vi "Receive.vi"(10 "MessageBuffer":T1, 11 "Clear?":bool) -> (2 "Receive":string[][](array[string]))   [LabVIEW 2020]
panel:
  out "error out":errorcluster caption="错误输出"
  in  "error in":errorcluster caption="错误输入"
  # "Receive"
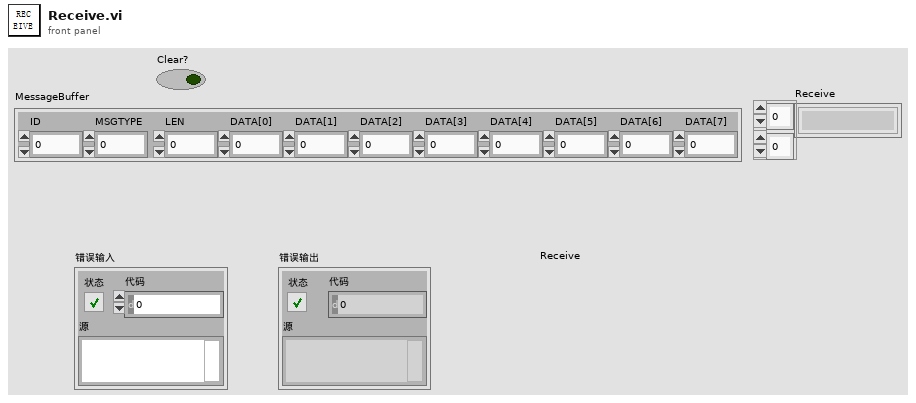
[diagram p1: front panel]
types:
  T1 = cluster{"ID":u32, "MSGTYPE":u8, "LEN":u8, "DATA[0]":u8, "DATA[1]":u8, "DATA[2]":u8, "DATA[3]":u8, "DATA[4]":u8, "DATA[5]":u8, "DATA[6]":u8, "DATA[7]":u8}
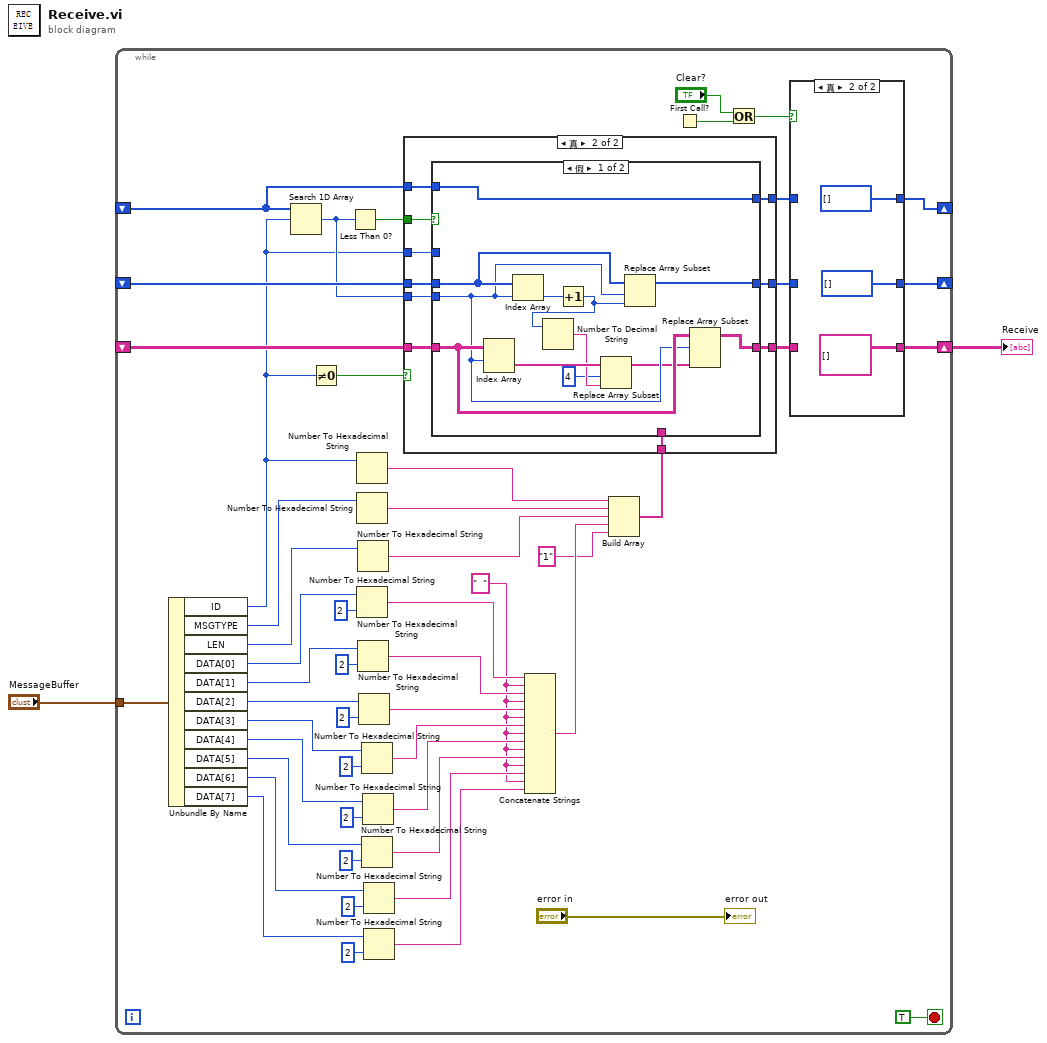
[diagram p0: block diagram]
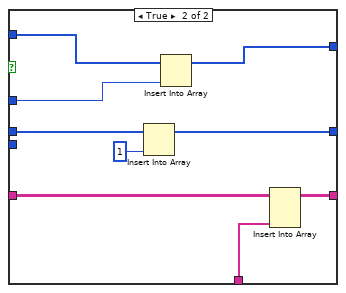
[diagram p3: hidden frame]
diagram:
  n1 = while {
    tunnel: "MessageBuffer" -> [w54]
    shift-right: [w20] -> _
    shift-left: _ -> [w6]
    shift-right: [w19] -> _
    shift-left: _ -> [w17]
    shift-right: [w14] -> w1
    shift-left: _ -> [w13]
    stop <- TRUE stop-if-true
    w27 = "  "
    n2 = Unbundle By Name(w54) -> ("ID"=w4:u32, "MSGTYPE"=w53:u8, "LEN"=w52:u8, "DATA[0]"=w51:u8, "DATA[1]"=w48:u8, "DATA[2]"=w46:u8, "DATA[3]"=w44:u8, "DATA[4]"=w42:u8, "DATA[5]"=w38:u8, "DATA[6]"=w37:u8, "DATA[7]"=w36:u8)
    n3 = Search 1D Array(1D array=w6, element=w4) -> (index of element=w15:i32)  [unwired: 1 in]
    n4 = Not Equal To 0?(x=w4) -> (x != 0?=w3:bool)
    n5 = Less Than 0?(x=w15) -> (x < 0?=w18:bool)
    n6 = Number To Hexadecimal String(2:w4) -> (0:w26:string)  [unwired: 1 in]
    n7 = Number To Hexadecimal String(2:w53) -> (0:w25:string)  [unwired: 1 in]
    n8 = Number To Hexadecimal String(1:i16 2 ("宽度(-)"), 2:w51) -> (0:w35:string)
    n9 = Number To Hexadecimal String(2:w52) -> (0:w24:string)  [unwired: 1 in]
    n10 = Number To Hexadecimal String(1:i16 2 ("宽度(-)"), 2:w48) -> (0:w34:string)
    n11 = Number To Hexadecimal String(1:i16 2 ("宽度(-)"), 2:w46) -> (0:w33:string)
    n12 = Number To Hexadecimal String(1:i16 2 ("宽度(-)"), 2:w44) -> (0:w32:string)
    n13 = Number To Hexadecimal String(1:i16 2 ("宽度(-)"), 2:w38) -> (0:w30:string)
    n14 = Number To Hexadecimal String(1:i16 2 ("宽度(-)"), 2:w42) -> (0:w31:string)
    n15 = Number To Hexadecimal String(1:i16 2 ("宽度(-)"), 2:w37) -> (0:w29:string)
    n16 = Number To Hexadecimal String(1:i16 2 ("宽度(-)"), 2:w36) -> (0:w28:string)
    n17 = Concatenate Strings(w35, w27, w34, w27, w33, w27, w32, w27, w31, w27, w30, w27, w29, w27, w28) -> (w23:string)
    n18 = Build Array(w26, w25, w24, w23, "1" ("元素")) -> (w11:string[])
    n19 = case shown="真" w3 {
      tunnel: w18 -> [_ w67]
      tunnel: w17 -> [w56 w66]
      tunnel: [w56 w65] -> w16
      tunnel: w15 -> [_ w64]
      tunnel: w13 -> [w55 w63]
      tunnel: [w55 w62] -> w12
      tunnel: w11 -> [_ w61]
      tunnel: w6 -> [w57 w60]
      tunnel: w4 -> [_ w59]
      tunnel: [w57 w58] -> w5
      frame False {
      }
      frame True {
        n20 = case shown="假" w67 {
          tunnel: w66 -> [w78 w88]
          tunnel: [w77 w87] -> w65
          tunnel: w64 -> [w74 _]
          tunnel: w63 -> [w75 w85]
          tunnel: [w73 w84] -> w62
          tunnel: w61 -> [_ w83]
          tunnel: w60 -> [w68 w82]
          tunnel: w59 -> [_ w81]
          tunnel: [w68 w80] -> w58
          frame False {
            n21 = Index Array(array=w75, index (row)=w74) -> (element=w72:string[])  [unwired: 1 in]
            n22 = Index Array(array=w78, index=w74) -> (element=w79:u32)
            n23 = Increment(x=w79) -> (x+1=w76:u32)
            n24 = Number To Decimal String(number=w76) -> (decimal integer string=w71:string)  [unwired: 1 in]
            n25 = Replace Array Subset(array=w72, new element=w71, index=4 ("索引")) -> (w69:string[])
            n26 = Replace Array Subset(array=w78, new element=w76, index=w74) -> (w77:u32[])
            n27 = Replace Array Subset(array=w75, new element=w69, index (row)=w74) -> (w73:string[][])  [unwired: 1 in]
          }
          frame True {
            n28 = Insert Into Array(array=w88, new element=u32 1 ("新元素/子数组")) -> (w87:u32[])  [unwired: 1 in]
            n29 = Insert Into Array(array=w82, new element=w81) -> (w80:u32[])  [unwired: 1 in]
            n30 = Insert Into Array(array=w85, new element=w83) -> (w84:string[][])  [unwired: 2 in]
          }
        }
      }
    }
    n31 = First Call?() -> (First Call?: T/F=w22:bool)
    n32 = Or(x="Clear?", y=w22) -> (x .or. y?=w7:bool)
    n33 = case shown="真" w7 {
      tunnel: [w91 u32[] [] ("ID")] -> w20
      tunnel: w5 -> [w91 _]
      tunnel: [w90 u32[] [] ("ID")] -> w19
      tunnel: w16 -> [w90 _]
      tunnel: [w89 string[][] []] -> w14
      tunnel: w12 -> [w89 _]
      frame False {
      }
      frame True {
      }
    }
    "error out" <- "error in"
  }
  "Receive" <- w1
